vi "JoyStick.vi"(8 "error in (no error)":errorcluster, 10 "On/Off":bool, 11 ".NET Refnum in":refnum<k24>) -> (0 "error out":errorcluster, 3 "controller out":refnum<k24>)   [LabVIEW 2016]
uses:
  C:/Users/TTUHEP/Documents/LabVIEW/Other Models/2010/Bin/Aerotech.A3200.dll
  Other Models/2010/Bin/Aerotech.A3200.dll
  Other Models/2010/Motion/AbortSingle.vi
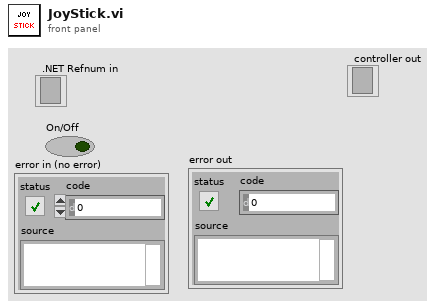
[diagram p1: front panel]
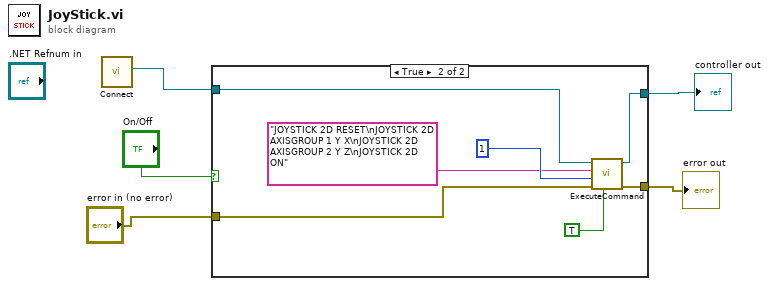
[diagram p0: block diagram]
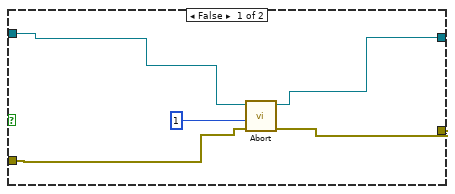
[diagram p2: hidden frame]
diagram:
  n1 = call "Connect.vi"() -> ("controller"=w1:refnum<k24>)  [unwired: 10 in, 1 out]
  n2 = case shown="True" "On/Off" {
    tunnel: w1 -> [w8 w16]
    tunnel: "error in (no error)" -> [w10 w13]
    tunnel: [w6 w12] -> w3
    tunnel: [w7 w11] -> w2
    frame False {
      n3 = call-poly "Abort.vi"("error in (no error)"=w10, "taskId"=1, "controller in"=w8) -> ("error out"=w6:errorcluster, "controller out"=w7:refnum<k24>)  [unwired: 7 in]
    }
    frame True {
      n4 = call "ExecuteCommand.vi"("return immediately"=TRUE, "error in (no error)"=w13, "taskId"=1, "Command Code"="JOYSTICK 2D RESET\nJOYSTICK 2D AXISGROUP 1 Y X\nJOYSTICK 2D AXISGROUP 2 Y Z\nJOYSTICK 2D ON", "controller in"=w16) -> ("error out"=w12:errorcluster, "controller out"=w11:refnum<k24>)  [unwired: 4 in, 1 out]
    }
  }
  "error out" <- w3
  "controller out" <- w2
